vi "Read All.vi"(8 "error in":errorcluster, 11 "VISA Refnum in":refnum<visa-resource-name>) -> (0 "error out":errorcluster, 2 "Final Output":string, 3 "VISA out":refnum<visa-resource-name>)   [LabVIEW 2018]
uses:
  <vilib>/Analysis/Matrix/Datatypes/RealMatrix.ctl
  <vilib>/regexp/Match Regular Expression.xnode
  <vilib>/Analysis/Matrix/NI_Matrix.lvlib
panel:
  out "concatenated string":string
  out "Channel Read as Matrix":T1
  out "before match":string
  out "whole match":string
  out "after match":string
  out "offset past match":i32
  out "read buffer":string
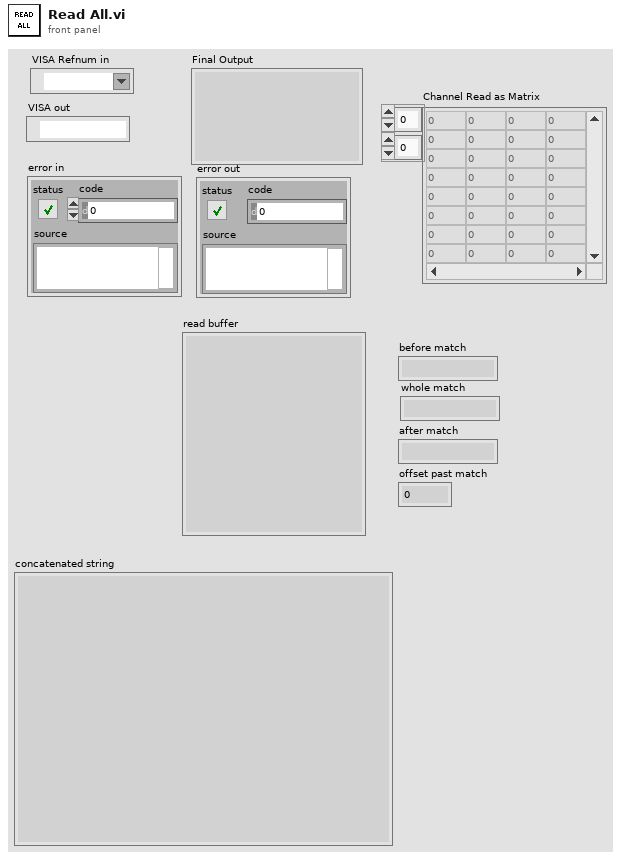
[diagram p1: front panel]
types:
  T1 = typedef "NI_Matrix.lvlib/RealMatrix.ctl" = dbl[][]
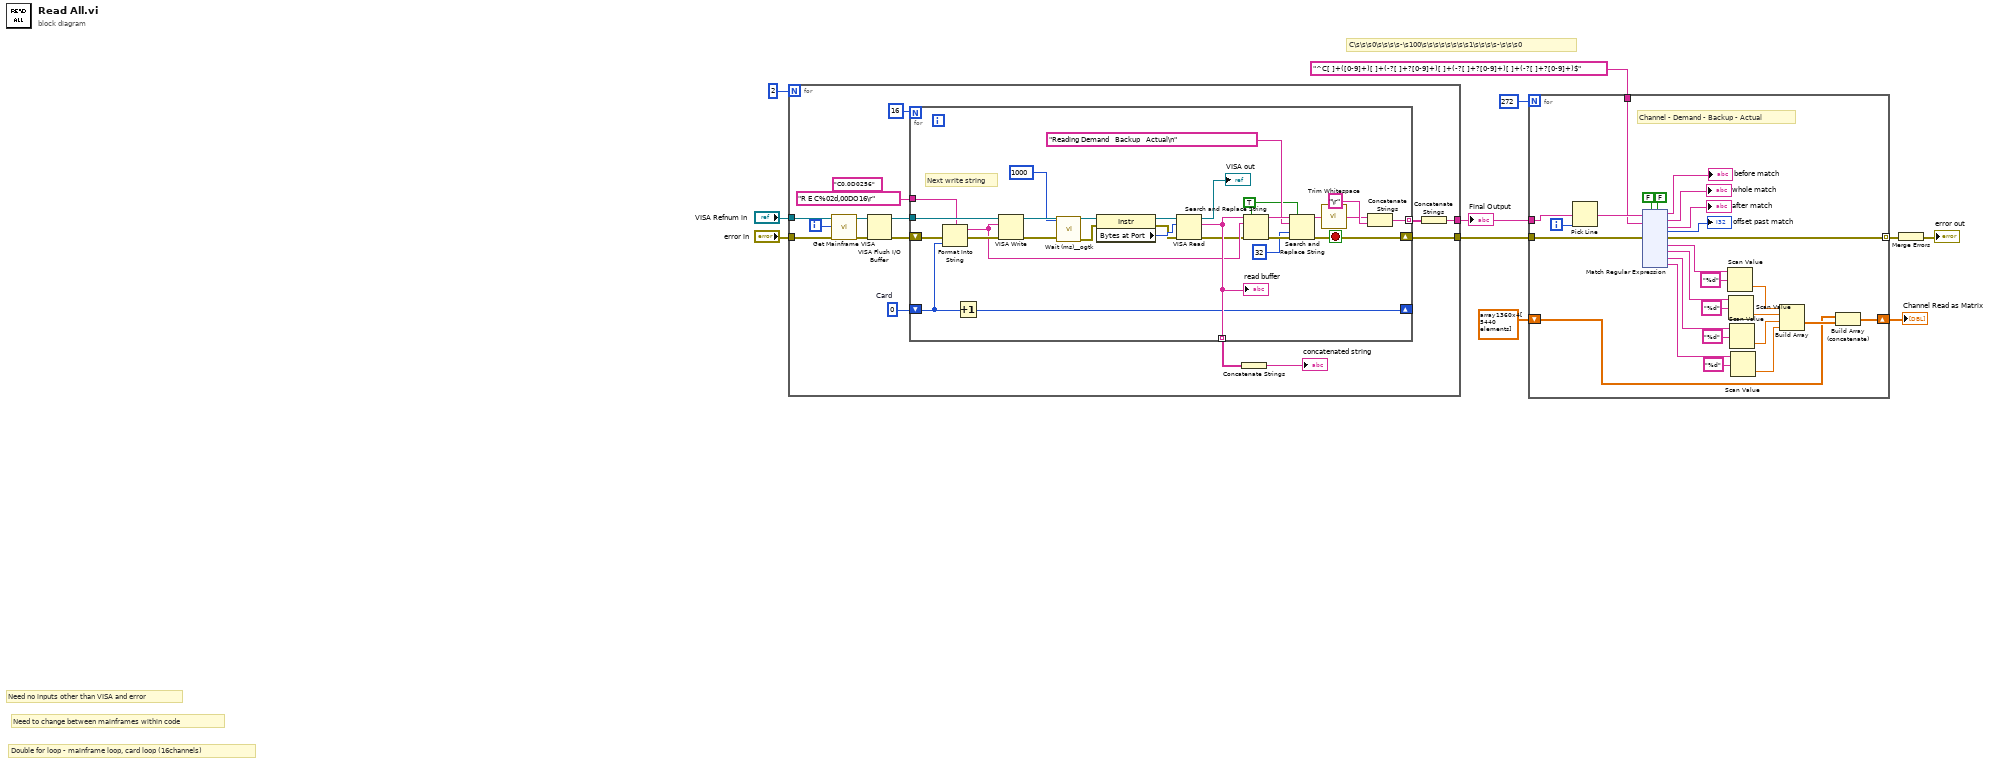
[diagram p0: block diagram]
diagram:
  # "C\\s\\s\\s0\\s\\s\\s\\s-\\s100\\s\\s\\s\\s\\s\\s\\s\\s1\\s\\s\\s\\s-\\s\\s\\s0"
  # "Double for loop - mainframe loop, card loop (16channels)"
  # "Need to change between mainframes within code"
  # "Need no inputs other than VISA and error"
  n1 = for {
    N: 2 -> [_]
    tunnel: "error in" -> [w23]
    tunnel: "VISA Refnum in" -> [w21]
    tunnel: [w14] -> w8
    tunnel: [w13] -> w5
    i -> [w20]
    (unwired) "C0,0D0256" ("C##,##DO###")
    w19 = 0  # Card
    n2 = call "Get Mainframe VISA.vi"("Error In"=w23, "Crate"=w20, "VISA In"=w21) -> ("Error Out"=w22:errorcluster, "VISA out"=w24:refnum<visa-resource-name>)  [unwired: 6 in, 1 out]
    n3 = VISA Flush I/O Buffer(VISA resource name=w24, error in (no error)=w22) -> (VISA resource name out=w25:refnum<visa-resource-name>, error out=w18:errorcluster)  [unwired: 1 in]
    n4 = for {
      N: 16 -> [_]
      tunnel: w25 -> [w53]
      tunnel: [w52] -> w16 mode=indexing
      shift-right: [w50] -> _
      shift-left: w19 -> [w51]
      shift-right: [w30] -> w13
      shift-left: w18 -> [w31]
      tunnel: [w28] -> w17 mode=indexing
      tunnel: "R E C%02d,00DO16\r" ("format string") -> [w27]
      stop <- w30 stop-if-true
      w32 = TRUE ("replace all? (F)")
      # "Next write string"
      n5 = Format Into String(format string=w27, error in=w31, w51) -> (resulting string=w39:string, error out=w49:errorcluster)  [unwired: 1 in]
      n6 = Increment(x=w51) -> (x+1=w50:i32)
      n7 = VISA Write(VISA resource name=w53, write buffer=w39, error in (no error)=w49) -> (VISA resource name out=w46:refnum<visa-resource-name>, error out=w48:errorcluster)  [unwired: 1 out]
      n8 = call <userlib>:"Wait (ms)__ogtk.vi"("error in (no error)"=w48, "milliseconds to wait"=u32 1000) -> ("error out"=w47:errorcluster)  [unwired: 8 in, 1 out]
      n9 = property class="Instr"(reference=w46, error in=w47) -> (reference out=w44:refnum<visa-resource-name>, error out=w43:errorcluster, "Bytes at Port"=w45:u32)
      n10 = VISA Read(VISA resource name=w44, byte count=w45, error in (no error)=w43) -> (VISA resource name out=→"VISA out":refnum<visa-resource-name>, read buffer=w52:string, error out=w38:errorcluster)  [unwired: 1 out]
      "read buffer" <- w52
      n11 = Search and Replace String(replace all?=w32, input string=w52, search string=w39, error in=w38) -> (result string=w37:string, error out=w36:errorcluster)  [unwired: 4 in, 2 out]
      n12 = Search and Replace String(replace all?=w32, input string=w37, search string="Reading Demand   Backup   Actual\n", offset=32 ("offset (0)"), error in=w36) -> (result string=w35:string, error out=w30:errorcluster)  [unwired: 3 in, 2 out]
      n13 = call <vilib>:"Trim Whitespace.vi"("string"=w35) -> ("trimmed string"=w29:string)  [unwired: 1 in]
      n14 = Concatenate Strings(w29, "\r" ("string")) -> (w28:string)
    }
    n15 = Concatenate Strings(w16) -> (→"concatenated string":string)
    n16 = Concatenate Strings(w17) -> (w14:string)
  }
  "Final Output" <- w8
  n17 = for {
    N: 272 -> [_]
    tunnel: w8 -> [w59]
    tunnel: "^C[ ]+([0-9]+)[ ]+(-?[ ]+?[0-9]+)[ ]+(-?[ ]+?[0-9]+)[ ]+(-?[ ]+?[0-9]+)$" -> [w58]
    tunnel: w5 -> [w57]
    tunnel: [w56] -> w4 mode=indexing
    shift-right: [w54] -> w1
    shift-left: T1 array1360x4[5440 elements] ("Channel Read as Matrix") -> [w55]
    i -> [w66]
    # "Channel - Demand - Backup - Actual"
    n18 = Pick Line(multi-line string=w59, line index=w66) -> (output string=w65:string)  [unwired: 1 in]
    n19 = xnode "Match Regular Expression"("input string"=w65, "regular expression"=w58, "error in"=w57, "ignore case? (F)"=FALSE, "multiline? (F)"=FALSE) -> ("before match"=→"before match":string, "whole match"=→"whole match":string, "after match"=→"after match":string, "offset past match"=→"offset past match":i32, "error out"=w56:errorcluster, "submatch 1"=w74:string, "submatch 2"=w69:string, "submatch 3"=w68:string, "submatch 4"=w67:string)  [unwired: 1 in]
    n20 = Scan Value(string=w74, format string="%d") -> (value=w64:dbl)  [unwired: 1 in, 1 out]
    n21 = Scan Value(string=w69, format string="%d") -> (value=w63:dbl)  [unwired: 1 in, 1 out]
    n22 = Scan Value(string=w68, format string="%d") -> (value=w62:dbl)  [unwired: 1 in, 1 out]
    n23 = Scan Value(string=w67, format string="%d") -> (value=w61:dbl)  [unwired: 1 in, 1 out]
    n24 = Build Array ("Build Matrix")(w64, w63, w62, w61) -> (w60:T1)
    n25 = Build Array (concatenate) ("Build Matrix")(w55, w60) -> (w54:T1)
  }
  "Channel Read as Matrix" <- w1
  n26 = Merge Errors(w4) -> (→"error out":errorcluster)
